vi "go_to_point.vi"(1 "error in":errorcluster, 2 "data":dbl[](array[numeric]) format="%0.2f") -> (0 "error out":errorcluster)   [LabVIEW 2013]
uses:
  <vilib>/DAQmx/write.llb/DAQmx Write (Analog 1D DBL NChan 1Samp).vi
  <vilib>/DAQmx/create/channels.llb/DAQmx Create Channel (AO-Voltage-Basic).vi
  <vilib>/DAQmx/miscellaneous.llb/DAQmx Fill In Error Info.vi
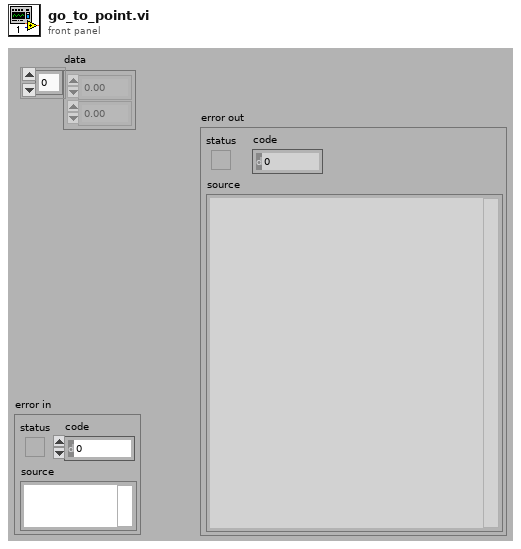
[diagram p1: front panel]
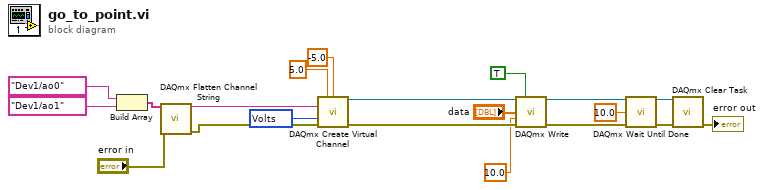
[diagram p0: block diagram]
diagram:
  w5 = 10348 items=["Volts"=10348, "From Custom Scale"=10065] ("units")
  n1 = Build Array(tag "Dev1/ao0" ("physical channels"), tag "Dev1/ao1" ("physical channels")) -> (w18:tag[])
  n2 = call <vilib>:"DAQmx Flatten Channel String.vi"("names in"=w18, "error in"="error in") -> ("names out"=w17:string, "error out"=w14:errorcluster)  [unwired: 12 in]
  n3 = call-poly <vilib>:"DAQmx Create Virtual Channel.vi"("maximum value"=5.0, "minimum value"=-5.0, "physical channels"=w17, "units"=w5, "error in"=w14) -> ("task out"=w9:refnum<k21>, "error out"=w8:errorcluster)  [unwired: 9 in]
  n4 = call-poly <vilib>:"DAQmx Write.vi"("task/channels in"=w9, "auto start"=TRUE, "data"="data", "timeout"=10.0, "error in"=w8) -> ("task out"=w3:refnum<k21>, "error out"=w2:errorcluster)  [unwired: 8 in, 1 out]
  n5 = call <vilib>:"DAQmx Wait Until Done.vi"("task/channels in"=w3, "timeout (sec)"=10.0, "error in"=w2) -> ("task out"=w12:refnum<k21>, "error out"=w13:errorcluster)  [unwired: 11 in]
  n6 = call <vilib>:"DAQmx Clear Task.vi"("task in"=w12, "error in"=w13) -> ("error out"=→"error out":errorcluster)  [unwired: 13 in]
